vi "Destroy User Event - Stop.vi"(8 "error in (no error)":errorcluster, 11 "User Events in":T1) -> (0 "error out":errorcluster)   [LabVIEW 2019, in "User Event - Stop.lvlib"]
doc: "Destroy the user event, even if there is an incoming error."
uses:
  User Event - Stop.lvlib
  controls/UserEvents_v2.ctl
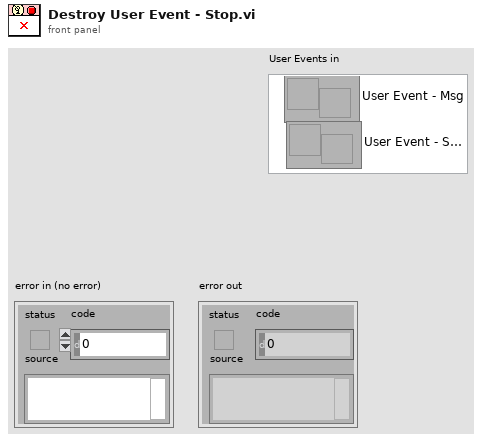
[diagram p1: front panel]
types:
  T1 = typedef "UserEvents_v2.ctl" = cluster{"User Event - Msg":refnum<user-event>, "User Event - Stop":refnum<user-event>}
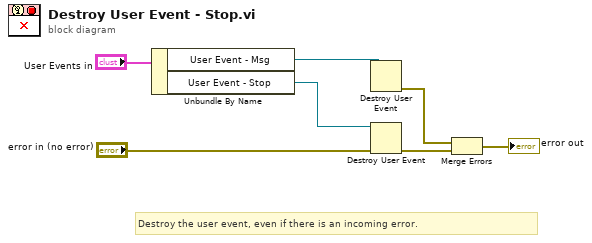
[diagram p0: block diagram]
diagram:
  # "Destroy the user event, even if there is an incoming error."
  n1 = Unbundle By Name("User Events in") -> ("User Event - Msg"=w3:refnum<user-event>, "User Event - Stop"=w1:refnum<user-event>)
  n2 = Destroy User Event(user event=w3) -> (error out=w2:errorcluster)  [unwired: 1 in]
  n3 = Destroy User Event(user event=w1, error in="error in (no error)") -> (error out=w7:errorcluster)
  n4 = Merge Errors(w2, w7) -> (→"error out":errorcluster)
